vi "Apply DSF Configuration to Node.vi"(8 "error in (no error)":errorcluster, 10 "File Path":path, 11 "Item Ref in":T1 format="%.0x") -> (0 "error out":errorcluster)   [LabVIEW 2017, in "Data Sharing Framework System Explorer.lvlib"]
uses:
  Data Sharing Framework System Explorer.lvlib
  <vilib>/NI Veristand/Custom Device API/Custom Device Item Ref.ctl
  <vilib>/NI VeriStand/Custom Device API/Custom Device API.lvlib
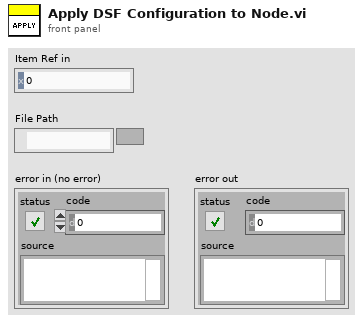
[diagram p1: front panel]
types:
  T1 = typedef "Custom Device API.lvlib/Custom Device Item Ref.ctl" = u64
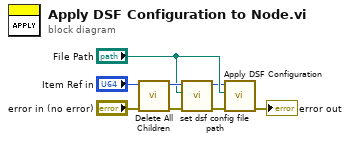
[diagram p0: block diagram]
diagram:
  n1 = call "Delete All Children.vi"("error in (no error)"="error in (no error)", "Item Ref in"="Item Ref in") -> ("error out"=w6:errorcluster, "Item Ref out"=w4:T1)  [unwired: 8 in]
  n2 = call "set dsf config file path.vi"("error in (no error)"=w6, "Path"="File Path", "Item Ref in"=w4) -> ("error out"=w1:errorcluster, "Item Ref out"=w2:T1)  [unwired: 7 in]
  n3 = call "Apply DSF Configuration.vi"("error in (no error)"=w1, "path"="File Path", "Item Ref in"=w2) -> ("error out"=→"error out":errorcluster)  [unwired: 8 in]
